vi "GT_CrdData.vi"(3 "crd":i16, 4 "fifo":i16, 5 "rtn_In":cluster{"rtn":i16, "Func":string}) -> (0 "fifo out":i16, 1 "crd out":i16, 2 "rtn_Out":cluster{"rtn":i16, "Func":string})   [LabVIEW 2014]
uses:
  VC6/gts.dll
panel:
  out "StringArray":string[](array[string])
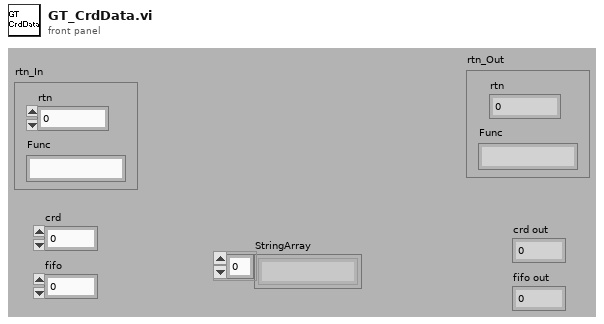
[diagram p1: front panel]
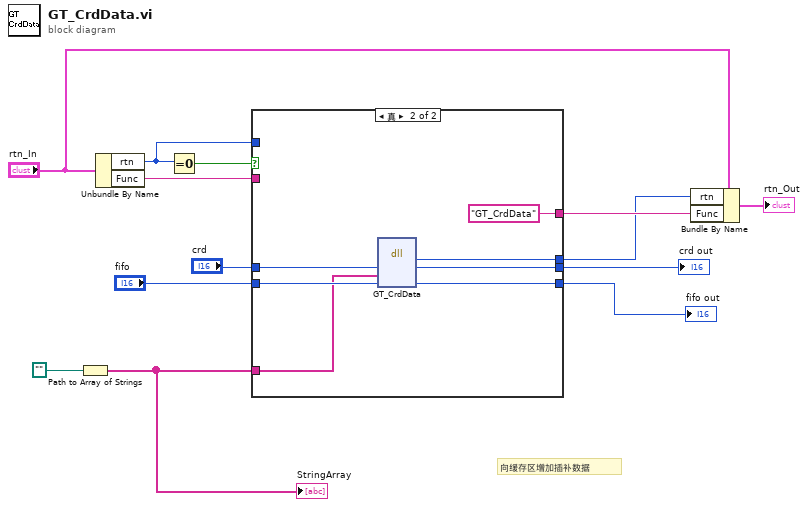
[diagram p0: block diagram]
diagram:
  # "向缓存区增加插补数据"
  n1 = Path to Array of Strings(0:path "") -> (2:w5:string[])  [unwired: 1 out]
  "StringArray" <- w5
  n2 = Unbundle By Name("rtn_In") -> ("rtn"=w7:i16, "Func"=w1:string)
  n3 = Equal To 0?(x=w7) -> (x = 0?=w13:bool)
  n4 = case shown="真" w13 {
    tunnel: "crd" -> [w15 w24]
    tunnel: "fifo" -> [w14 w23]
    tunnel: [w17 "GT_CrdData" ("Func")] -> w8
    tunnel: w7 -> [w16 _]
    tunnel: w5 -> [_ w21]
    tunnel: [w16 w20] -> w4
    tunnel: [w15 w19] -> w3
    tunnel: [w14 w18] -> w2
    tunnel: w1 -> [w17 _]
    frame False {
    }
    frame True {
      n5 = dll-call lib="PTH2Fabs DNewGTS AC-800LWin7版源程序-20170926gts85VC6gts.dll" fn="GT_CrdData"("crd"=w24, "pCrdData"=w21, "fifo"=w23) -> ("rtn"=w20:i16, "crd"=w19:i16, "fifo"=w18:i16)  [unwired: 4 in, 2 out]
    }
  }
  "crd out" <- w3
  "fifo out" <- w2
  n6 = Bundle By Name(cluster="rtn_In", "rtn"=w4, "Func"=w8) -> (→"rtn_Out":cluster{"rtn":i16, "Func":string})
